vi "Initialize Scalar Datatypes and Refs.vi"(8 "error in (no error)":errorcluster, 10 "Registers":T1[](array[typedef]) {"Register"."Data Type" format="%.0x"}, 11 "FPGA Ref":refnum<k20>) -> (0 "error out":errorcluster, 2 "Registers Ref":T5[](array[typedef]) {"Data Type" format="%.0x"}, 3 "FPGA Ref":refnum<k20>)   [LabVIEW 2015, in "FPGA Addon Engine.lvlib"]
uses:
  FPGA Addon Engine.lvlib
  Types/Register Settings.ctl
  Shared/Data Type.ctl
  Shared/Scalar Type.ctl
  Shared/Compiled.RegisterSettings.ctl
  Shared/Register Information.ctl
  Shared/FPGA Addon Shared.lvlib
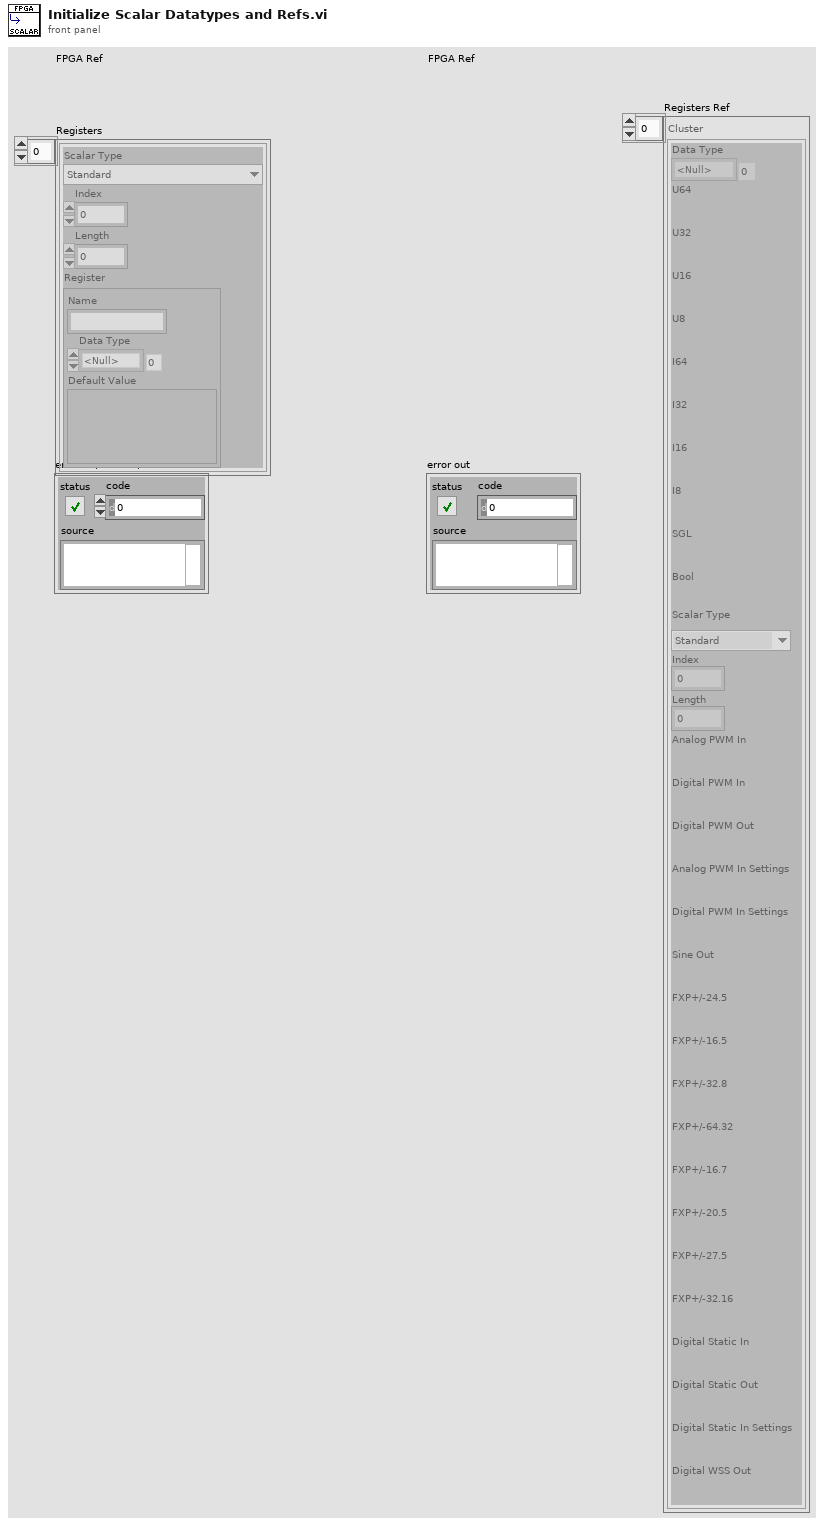
[diagram p1: front panel]
types:
  T1 = typedef "FPGA Addon Shared.lvlib/Compiled.RegisterSettings.ctl" = cluster{"Scalar Type":T2, "Index":i32, "Length":i32, "Register":T3}
  T2 = typedef "FPGA Addon Shared.lvlib/Scalar Type.ctl" = enum16{"Standard", "Bitpacked"}
  T3 = typedef "FPGA Addon Shared.lvlib/Register Information.ctl" = cluster{"Name":string, "Data Type":T4, "Default Value":variant}
  T4 = typedef "FPGA Addon Shared.lvlib/Data Type.ctl" = enum8{"<Null>", "I8", "I16", "I32", "I64", "U8", "U16", "U32", "U64", "SGL", "Boolean", "Analog PWM In Settings", "Analog PWM In", "Digital PWM In Settings", "Digital PWM In", "Digital PWM Out", "Sine Out", "FXP+/-24.5", "FXP+/-16.5", "FXP+/-32.8", "FXP+/-64.32", "FXP+/-16.7", "FXP+/-20.5", "FXP+/-27.5", "FXP+/-32.16", "Digital Static In", "Digital Static Out", "Digital Static In Settings", "Digital WSS Out"}
  T5 = typedef "FPGA Addon Engine.lvlib/Register Settings.ctl" = cluster{"Data Type":T4, "U64":refnum<k20>, "U32":refnum<k20>, "U16":refnum<k20>, "U8":refnum<k20>, "I64":refnum<k20>, "I32":refnum<k20>, "I16":refnum<k20>, "I8":refnum<k20>, "SGL":refnum<k20>, "Bool":refnum<k20>, "Scalar Type":T2, "Index":i32, "Length":i32, "Analog PWM In":refnum<k20>, "Digital PWM In":refnum<k20>, "Digital PWM Out":refnum<k20>, "Analog PWM In Settings":refnum<k20>, "Digital PWM In Settings":refnum<k20>, "Sine Out":refnum<k20>, "FXP+/-24.5":refnum<k20>, "FXP+/-16.5":refnum<k20>, "FXP+/-32.8":refnum<k20>, "FXP+/-64.32":refnum<k20>, "FXP+/-16.7":refnum<k20>, "FXP+/-20.5":refnum<k20>, "FXP+/-27.5":refnum<k20>, "FXP+/-32.16":refnum<k20>, "Digital Static In":refnum<k20>, "Digital Static Out":refnum<k20>, "Digital Static In Settings":refnum<k20>, "Digital WSS Out":refnum<k20>}
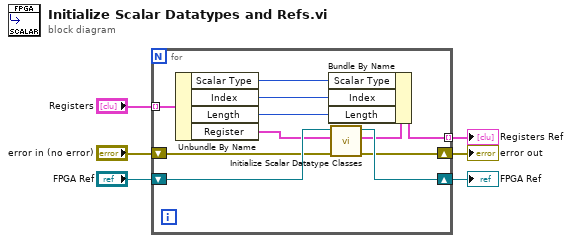
[diagram p0: block diagram]
diagram:
  n1 = for {
    shift-right: [w16] -> w4
    shift-left: "FPGA Ref" -> [w17]
    tunnel: [w14] -> w6 mode=indexing
    tunnel: "Registers" -> [w13] mode=indexing
    shift-right: [w7] -> w2
    shift-left: "error in (no error)" -> [w8]
    n2 = Unbundle By Name(w13) -> ("Scalar Type"=w9:T2, "Index"=w10:i32, "Length"=w11:i32, "Register"=w12:T3)
    n3 = call "Initialize Scalar Datatype Classes.vi"("error in (no error)"=w8, "Register"=w12, "FPGA Ref"=w17) -> ("error out"=w7:errorcluster, "Register"=w15:T5, "FPGA Ref"=w16:refnum<k20>)  [unwired: 6 in]
    n4 = Bundle By Name(cluster=w15, "Scalar Type"=w9, "Index"=w10, "Length"=w11) -> (w14:T5)
  }
  "error out" <- w2
  "Registers Ref" <- w6
  "FPGA Ref" <- w4
